vi "Path Notation End Name.vi"(11 "Item Path":string) -> (0 "Is Array":bool, 1 "Number of Paths":i32, 2 "<JSON>End Name":string)   [LabVIEW 2017, in "JSONtext.lvlib"]
uses:
  JSONtext.lvlib
  Advance past whitespace.vi
  Match Pattern.vi
  support/Quote and Escape JSON string.vi
  Advance past String.vi
  String Subset.vi
  Advance past whitespace and comma.vi
  <vilib>/JDP Science/JDP Science Common Utilities/Trim Whitespace__JDP.vi
  support/quote and escape json string 2.vi
  Parsing Error.vi
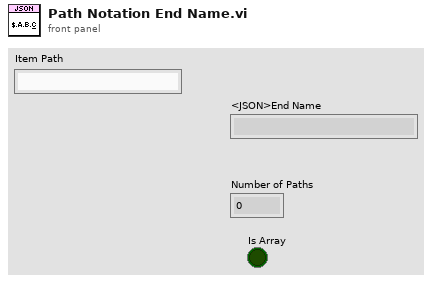
[diagram p1: front panel]
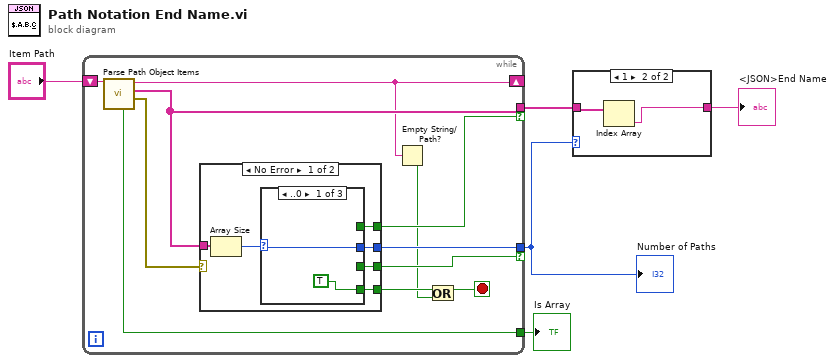
[diagram p0: block diagram]
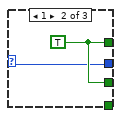
[diagram p2: hidden frame]
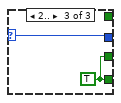
[diagram p3: hidden frame]
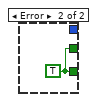
[diagram p4: hidden frame]
diagram:
  n1 = while {
    shift-right: [w9] -> _
    shift-left: "Item Path" -> [w16]
    tunnel: [w15] -> w3 if=w14
    tunnel: [w12] -> w2 if=w11
    tunnel: [w6] -> w1
    stop <- w8 stop-if-true
    n2 = call "Parse Path Object Items.vi"("Path with leading Object element"=w16) -> ("error out"=w10:errorcluster, "<JSON>items names"=w15:string[], "Rest or Path"=w9:string, "Is Array"=w6:bool)  [unwired: 7 in]
    n3 = case shown="No Error" w10 {
      tunnel: w15 -> [w22 _]
      tunnel: [w20 _] -> w14
      tunnel: [w19 w29] -> w13
      tunnel: [w18 _] -> w12
      tunnel: [w17 w29] -> w11
      frame No Error {
        n4 = Array Size(array=w22) -> (size(s)=w21:i32)
        n5 = case shown="..0" w21 {
          selector: w21 -> [w23 w25 w27]
          tunnel: [_ w26 _] -> w20
          tunnel: [TRUE _ w28] -> w19
          tunnel: [w23 w25 w27] -> w18
          tunnel: [_ w26 w28] -> w17
          frame ..0 {
          }
          frame 1 {
            w26 = TRUE
          }
          frame 2.. {
            w28 = TRUE
          }
        }
      }
      frame Error {
        w29 = TRUE
      }
    }
    n6 = Empty String/Path?(string/path=w9) -> (empty?=w7:bool)
    n7 = Or(x=w13, y=w7) -> (x .or. y?=w8:bool)
  }
  "Number of Paths" <- w2
  "Is Array" <- w1
  n8 = case shown="1" w2 {
    tunnel: w3 -> [_ w31]
    tunnel: [_ w30] -> w4
    frame Default {
    }
    frame 1 {
      n9 = Index Array(array=w31) -> (element=w30:string)  [unwired: 1 in]
    }
  }
  "<JSON>End Name" <- w4
